vi "利用数据队列的错误退出多线程.vi"(0 "退出":T1) -> (1 "队列输出":refnum<queue>, 2 "错误输出":errorcluster, 3 "数值":i32)   [LabVIEW 2019]
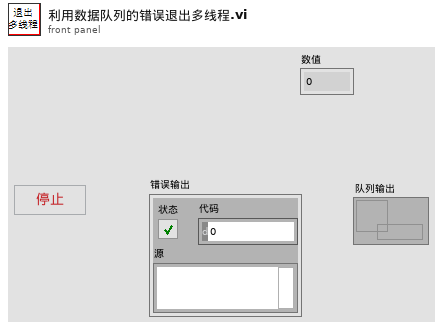
[diagram p1: front panel]
types:
  T1 = typedef "控件 1.ctl" = bool
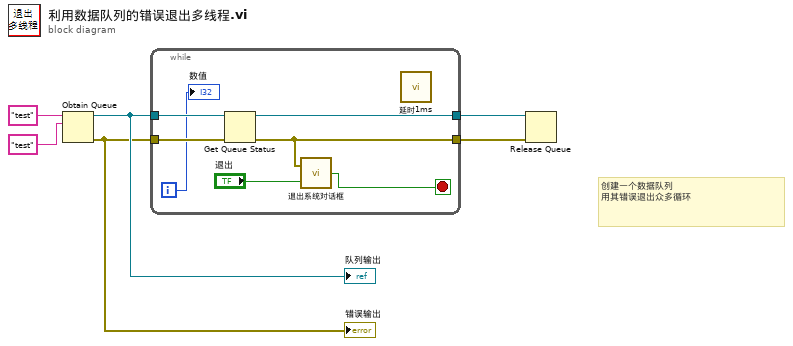
[diagram p0: block diagram]
diagram:
  # "创建一个数据队列\n用其错误退出众多循环"
  n1 = Obtain Queue(name (unnamed)="test" ("名称（未命名）"), element data type="test" ("名称（未命名）")) -> (queue out=w2:refnum<queue>, error out=w1:errorcluster)  [unwired: 3 in, 1 out]
  "错误输出" <- w1
  "队列输出" <- w2
  n2 = while {
    tunnel: w2 -> [w13]
    tunnel: w1 -> [w12]
    tunnel: [w11] -> w4
    tunnel: [w8] -> w3
    i -> [w7]
    stop <- w9 stop-if-true
    n3 = Get Queue Status(queue=w13, error in (no error)=w12) -> (queue out=w11:refnum<queue>, error out=w8:errorcluster)  [unwired: 1 in, 6 out]
    n4 = call "退出系统对话框.vi"("退出"="退出", "error in (no error)"=w8) -> ("T/F"=w9:bool)
    n5 = call "延时1ms.vi"() -> ()  [unwired: 12 in]
    "数值" <- w7
  }
  n6 = Release Queue(queue=w4, error in (no error)=w3) -> ()  [unwired: 1 in, 3 out]
